vi "MessungKommutierungskurve.vi"(0 "Spannungs Abweichung":dbl=5.0, 1 "maximale Spannung FG":dbl=10.0, 2 "Frequenz (1000 Hz)":dbl=1000.0, 3 "Messpunkte Oszi (6000)":i32=6000, 5 "VISA Name OZ In (OZ)":refnum<visa-resource-name>="USB0::0x0957::0x179B::MY54313507::INSTR", 6 "VISA Name FG in":refnum<visa-resource-name>="USB0::0x0957::0x0407::MY44043889::INSTR", 7 "error in":errorcluster, 8 "Faktor 2":dbl, 10 "Faktor 1":dbl, 12 "Anzahl Messpunkte Neukurve":i8=16 min=10 max=30 step=1, 14 "minimale Spannung FG":dbl) -> (21 "Output B Array":dbl[](array[numeric]), 22 "Output H Array":dbl[](array[numeric]), 25 "VISA Name OZ Out":refnum<visa-resource-name>="USB0::0x0957::0x179B::MY54313507::INSTR", 26 "VISA Name FG out":refnum<visa-resource-name>, 27 "error out":errorcluster)   [LabVIEW 2016]
uses:
  <instrlib>/Agilent 33XXX Series/Agilent 33XXX Series.lvlib
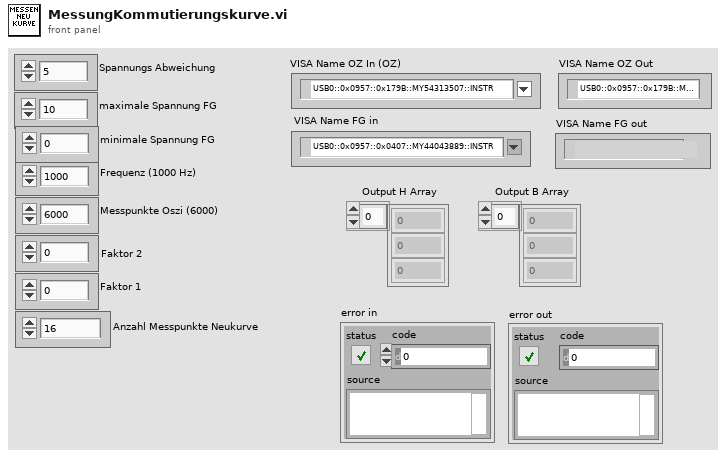
[diagram p1: front panel]
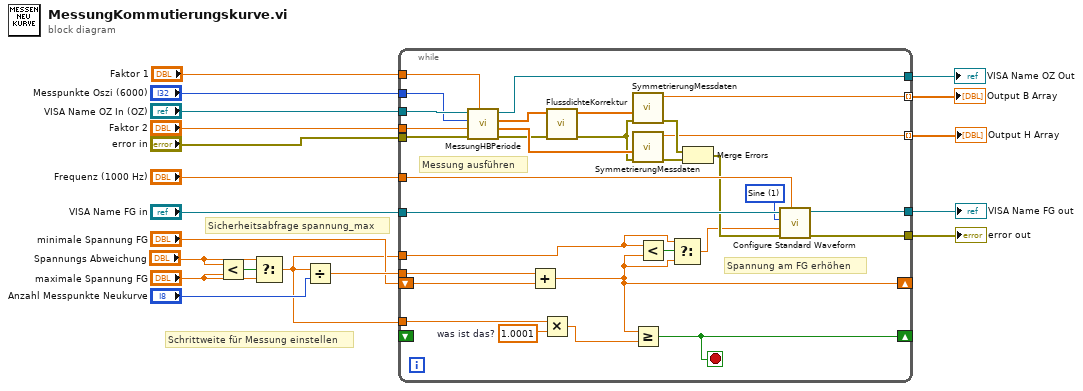
[diagram p0: block diagram]
diagram:
  # "Sicherheitsabfrage spannung_max"
  # "Schrittweite für Messung einstellen"
  n1 = Less?(x="Spannungs Abweichung", y="maximale Spannung FG") -> (x < y?=w19:bool)
  n2 = Select(t="Spannungs Abweichung", s=w19, f="maximale Spannung FG") -> (s? t:f=w3:dbl)
  n3 = Divide(x=w3, y="Anzahl Messpunkte Neukurve") -> (x/y=w7:dbl)
  n4 = while {
    tunnel: w7 -> [w48]
    tunnel: w3 -> [w47]
    tunnel: "error in" -> [w38]
    tunnel: "VISA Name FG in" -> [w43]
    tunnel: [w46] -> w17
    tunnel: [w45] -> w16
    tunnel: [w27] -> w2 mode=indexing
    tunnel: [w26] -> w1 mode=indexing
    tunnel: "VISA Name OZ In (OZ)" -> [w39]
    tunnel: "Faktor 1" -> [w33]
    tunnel: "Frequenz (1000 Hz)" -> [w44]
    tunnel: "Faktor 2" -> [w34]
    tunnel: "Messpunkte Oszi (6000)" -> [w37]
    shift-right: [w29] -> _
    shift-left: "minimale Spannung FG" -> [w40]
    tunnel: [w36] -> w6
    shift-right: [w25] -> _
    shift-left: _ -> [_]
    tunnel: w3 -> [w24]
    stop <- w25 stop-if-true
    w42 = u16 1 items=["DC", "Sine", "Square", "Triangle", "Ramp", "Pulse", "Noise", "Sinc", "Negative Ramp", "Exponential Rise", "Exponential Fall", "Cardiac"] ("Waveform Function (1: Sine)")
    w49 = 1.0001  # was ist das?
    # "Messung ausführen"
    # "Spannung am FG erhöhen"
    n5 = call "MessungHBPeriode.vi"("Faktor 1"=w33, "Error_in"=w38, "Faktor2 (1)"=w34, "Anzahl der Messpunkte"=w37, "VISA Name OZ in(OZ)"=w39) -> ("Error_out"=w23:errorcluster, "H-Messdaten einer periode"=w35:dbl[], "B-Messdaten einer periode"=w21:dbl[], "VISA Name OZ out(OZ)"=w36:refnum<visa-resource-name>)  [unwired: 3 in]
    n6 = Add(x=w48, y=w40) -> (x+y=w29:dbl)
    n7 = Multiply(x=w47, y=w49) -> (x*y=w50:dbl)
    n8 = call "FlussdichteKorrektur.vi"("error in"=w23, "B-Array in"=w21) -> ("error out"=w22:errorcluster, "B-Array out"=w20:dbl[])  [unwired: 8 in]
    n9 = call "SymmetrierungMessdaten.vi"("error in"=w22, "Input Array"=w20) -> ("error out"=w31:errorcluster, "xmax"=w27:dbl)  [unwired: 3 in, 3 out]
    n10 = call "SymmetrierungMessdaten.vi"("error in"=w22, "Input Array"=w35) -> ("error out"=w32:errorcluster, "xmax"=w26:dbl)  [unwired: 3 in, 3 out]
    n11 = Greater Or Equal?(x=w29, y=w50) -> (x >= y?=w25:bool)
    n12 = Less?(x=w24, y=w29) -> (x < y?=w30:bool)
    n13 = Select(t=w24, s=w30, f=w29) -> (s? t:f=w28:dbl)
    n14 = Merge Errors(w31, w32) -> (w41:errorcluster)
    n15 = call <instrlib>:"Configure Standard Waveform.vi"("Frequency (1000 Hz)"=w44, "error in (no error)"=w41, "Amplitude (1)"=w28, "Waveform Function (1: Sine)"=w42, "VISA resource name"=w43) -> ("error out"=w45:errorcluster, "VISA resource name out"=w46:refnum<visa-resource-name>)  [unwired: 5 in]
  }
  "error out" <- w16
  "VISA Name FG out" <- w17
  "Output B Array" <- w2
  "Output H Array" <- w1
  "VISA Name OZ Out" <- w6
